vi "reshape_mcs_spectra.vi"(8 "MCS Parameters":T1={"Scan Length (Bins)"=64.0, "Dwell Time (s)"=1e-07, "Gate Channel Settings"={"Threshold (V)"=0.0, "Edge"=enum."Falling", "Input Impedence"=enum."1k Ohm"}, "Trig Channel Settings"={"Threshold (V)"=0.0, "Edge"=enum."Falling", "Input Impedence"=enum."1k Ohm"}, "Input 1 Settings"={"Threshold (V)"=0.0, "Edge"=enum."Falling", "Input Impedence"=enum."1k Ohm"}, "Input 2 Settings"={"Threshold (V)"=0.0, "Edge"=enum."Falling", "Input Impedence"=enum."1k Ohm"}, "Number of Sweeps"=0, "Number of Sequential Cycles"=0.0, "Number of Sequences"=0.0, "Sweep Preset"=FALSE, "Sequential Mode"=FALSE, "DAC 1 Ramp Settings"={"Ramp Mode"=enum."Fixed", "Ramp Start Value (V)"=0.0, "Ramp Length (Steps)"=1, "Step Width (bins)"=0, "Step Size (V)"=0.0}, "DAC 2 Output (V)"=0.0, "SYNC Output"=enum."40 MHz Clock", "ROI Min"=0, "ROI Max"=1, "Dual MCS Mode"=FALSE, "DAC 2 Toggle"=FALSE, "MCS on/off"=FALSE, "ROI Max 2"=1, "ROI Min 2"=0, "Sum ROI Only"=FALSE, "Use ROI For \nEach Loop"=FALSE} {"ROI Max 2" min=1; "ROI Min 2" min=0; "ROI Max" min=1; "ROI Min" min=0; "DAC 2 Output (V)" min=-10.0 max=10.0 step=0.00488; "DAC 1 Ramp Settings"."Step Size (V)" min=0.0 max=10.0 step=0.00244 format="%#_4g"; "DAC 1 Ramp Settings"."Step Width (bins)" min=1; "DAC 1 Ramp Settings"."Ramp Length (Steps)" min=1; "DAC 1 Ramp Settings"."Ramp Start Value (V)" min=0.0 max=10.0 step=0.00244; "Number of Sweeps" min=0 format="%.0p"; "Input 2 Settings"."Threshold (V)" min=-2.5 max=2.5 step=0.001; "Input 1 Settings"."Threshold (V)" min=-2.5 max=2.5 step=0.001; "Trig Channel Settings"."Threshold (V)" min=-2.5 max=2.5 step=0.001; "Gate Channel Settings"."Threshold (V)" min=-2.5 max=2.5 step=0.001; "Dwell Time (s)" min=1e-07 step=2.5e-08 format="%#_6p"; "Scan Length (Bins)" min=64.0 max=524288.0 format="%#_7f"}, 9 "Spectrum Length":i32, 10 "Data":u32[](array[numeric])) -> (2 "2d Data":u32[][](array[numeric]))   [LabVIEW 2015]
uses:
  Controls/MCS/mcs_control_panel.ctl
  Controls/MCS/mcs_channel.ctl
  Controls/MCS/ramp_control.ctl
panel:
  out "Waveform Graph":u32[](graph)
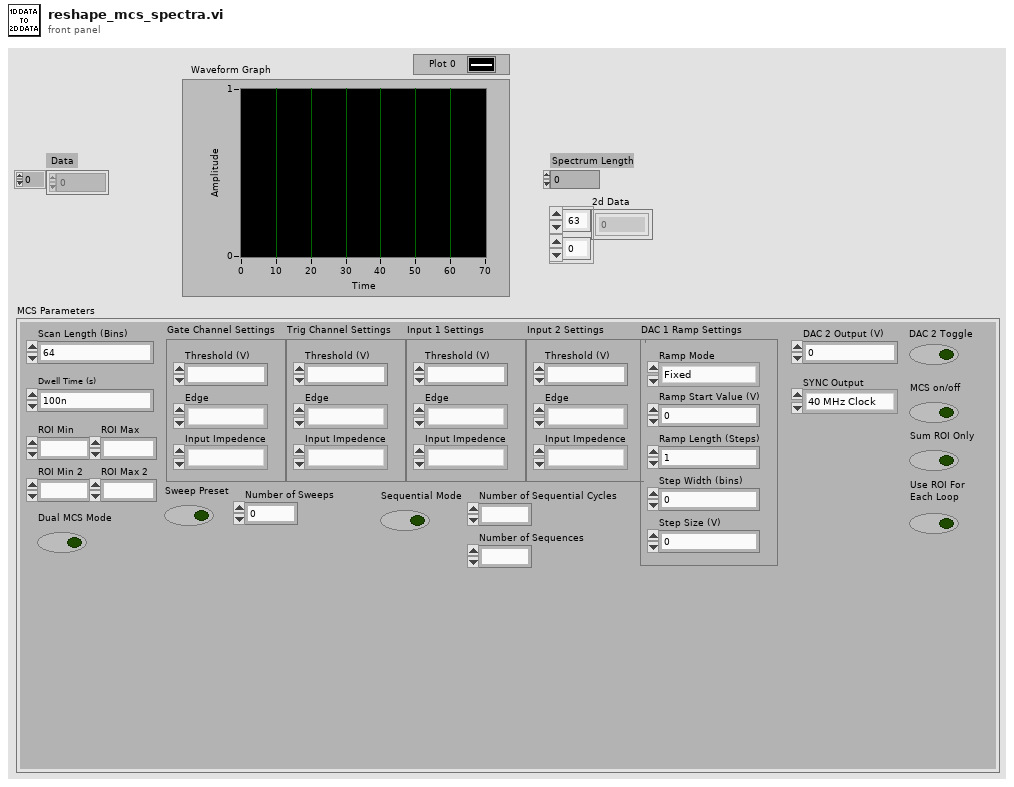
[diagram p1: front panel]
types:
  T1 = typedef "mcs_control_panel.ctl" = cluster{"Scan Length (Bins)":dbl, "Dwell Time (s)":dbl, "Gate Channel Settings":T2, "Trig Channel Settings":T2, "Input 1 Settings":T2, "Input 2 Settings":T2, "Number of Sweeps":i32, "Number of Sequential Cycles":dbl, "Number of Sequences":dbl, "Sweep Preset":bool, "Sequential Mode":bool, "DAC 1 Ramp Settings":T3, "DAC 2 Output (V)":dbl, "SYNC Output":enum16{"40 MHz Clock", "Gate Disc Signal", "Trigger Disc Signal", "Counter 1 Disc Signal", "Counter 2 Disc Signal", "Definitely Not Used", "Not Used", "1 kHz Signal", "Also Not Used", "MCS On/Off", "End of Time Bin", "Ramp Increment Trig", "Step Count Trigger", "'GO'-Line", "Ramp Down Trigger", "Logic 1"}, "ROI Min":i32, "ROI Max":i32, "Dual MCS Mode":bool, "DAC 2 Toggle":bool, "MCS on/off":bool, "ROI Max 2":i32, "ROI Min 2":i32, "Sum ROI Only":bool, "Use ROI For \nEach Loop":bool}
  T2 = typedef "mcs_channel.ctl" = cluster{"Threshold (V)":dbl, "Edge":enum16{"Falling", "Rising"}, "Input Impedence":enum16{"1k Ohm", "50 Ohm"}}
  T3 = typedef "ramp_control.ctl" = cluster{"Ramp Mode":enum16{"Fixed", "Triangle", "Sawtooth"}, "Ramp Start Value (V)":dbl, "Ramp Length (Steps)":i32, "Step Width (bins)":i32, "Step Size (V)":dbl}
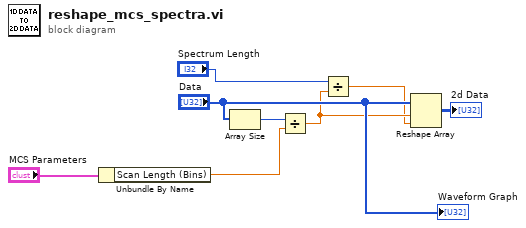
[diagram p0: block diagram]
diagram:
  n1 = Unbundle By Name("MCS Parameters") -> ("Scan Length (Bins)"=w5:dbl)
  n2 = Array Size(array="Data") -> (size(s)=w8:i32)
  n3 = Divide(x=w8, y=w5) -> (x/y=w2:dbl)
  n4 = Divide(x="Spectrum Length", y=w2) -> (x/y=w1:dbl)
  n5 = Reshape Array("Data", w2, w1) -> (→"2d Data":u32[][])
  "Waveform Graph" <- "Data"
